vi "p2 - caja fuerte.vi"() -> ()   [LabVIEW 2021]
uses:
  p2 - strongbox.ctl
  p2 - states.ctl
  <vilib>/DAQmx/write.llb/DAQmx Write (Analog DBL 1Chan 1Samp).vi
  <vilib>/DAQmx/read.llb/DAQmx Read (Counter DBL 1Chan 1Samp).vi
  <vilib>/DAQmx/miscellaneous.llb/DAQmx Fill In Error Info.vi
panel:
  in  "stop":bool
  out "turns IRT":dbl format="%0.2f"
  out "turns":i32
  out "direction":bool
  out "password":i32[](array[numeric])
  in  "clean":bool
  in  "unlock":bool
  in  "Knob":i32(knob)=1 scale=1.0..100.0
  out "Boolean":T1
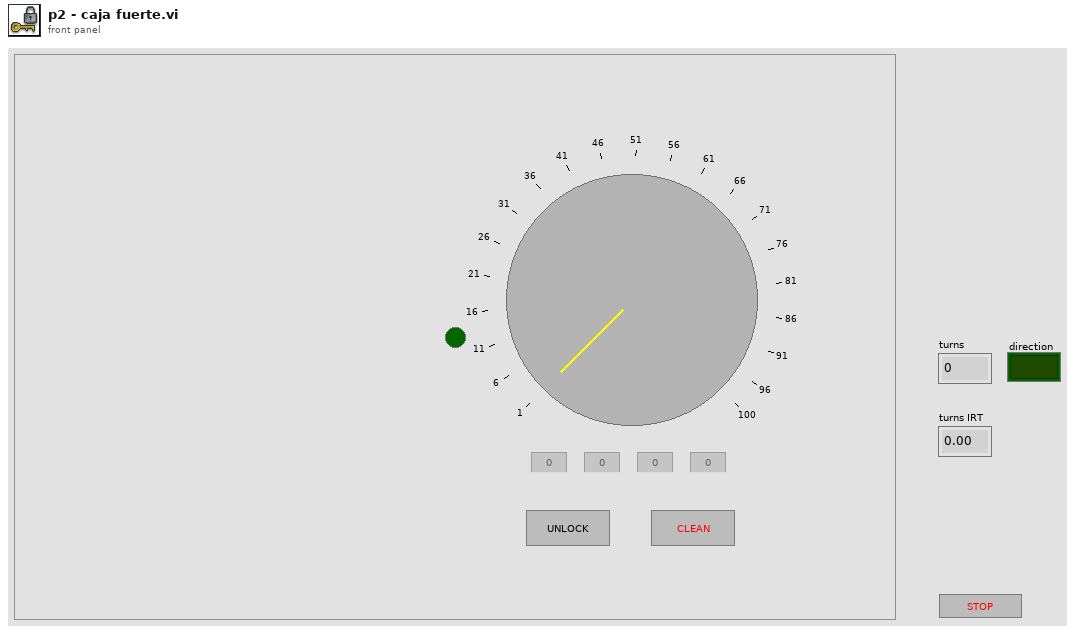
[diagram p1: front panel]
types:
  T1 = typedef "p2 - strongbox.ctl" = bool
  T2 = typedef "p2 - states.ctl" = enum16{"knob", "motor", "animation"}
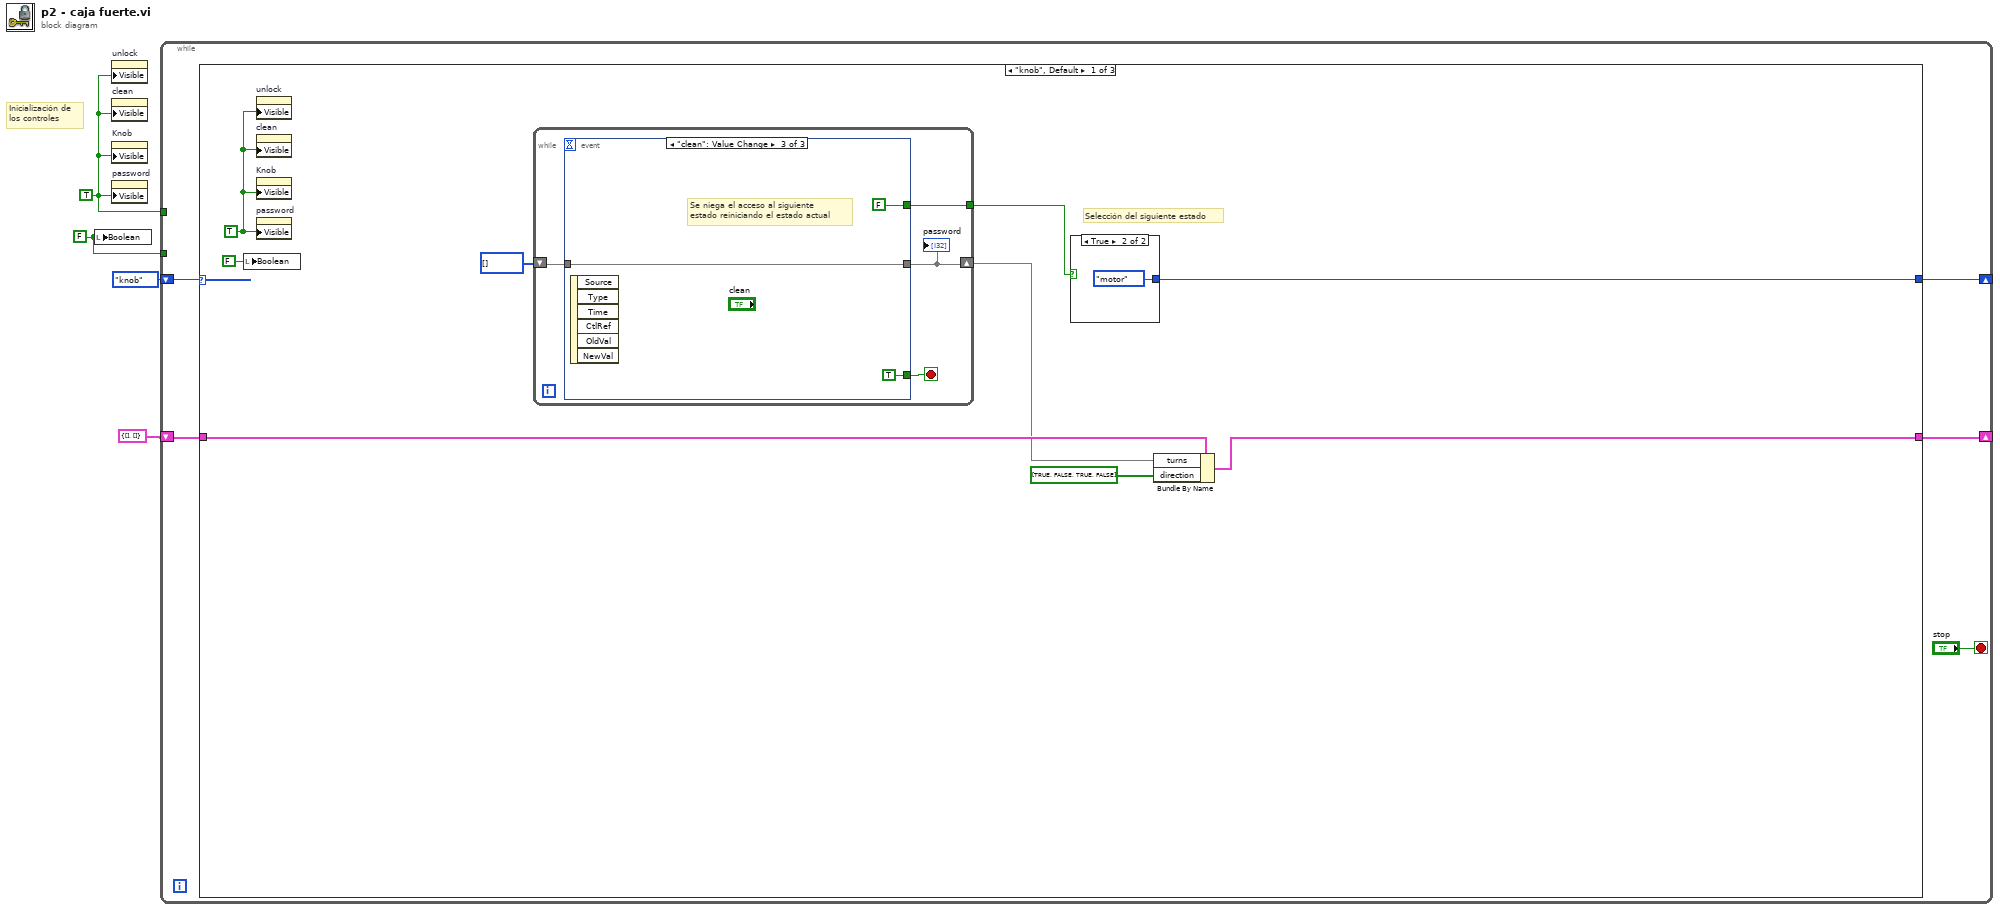
[diagram p0: block diagram]
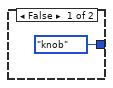
[diagram p2: hidden frame]
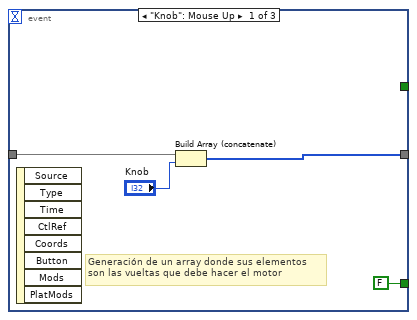
[diagram p3: hidden frame]
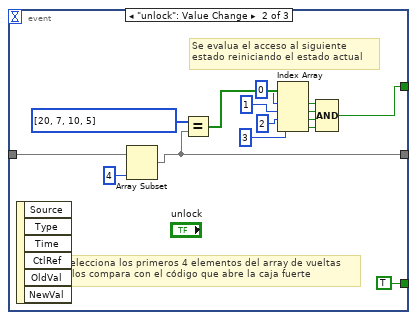
[diagram p4: hidden frame]
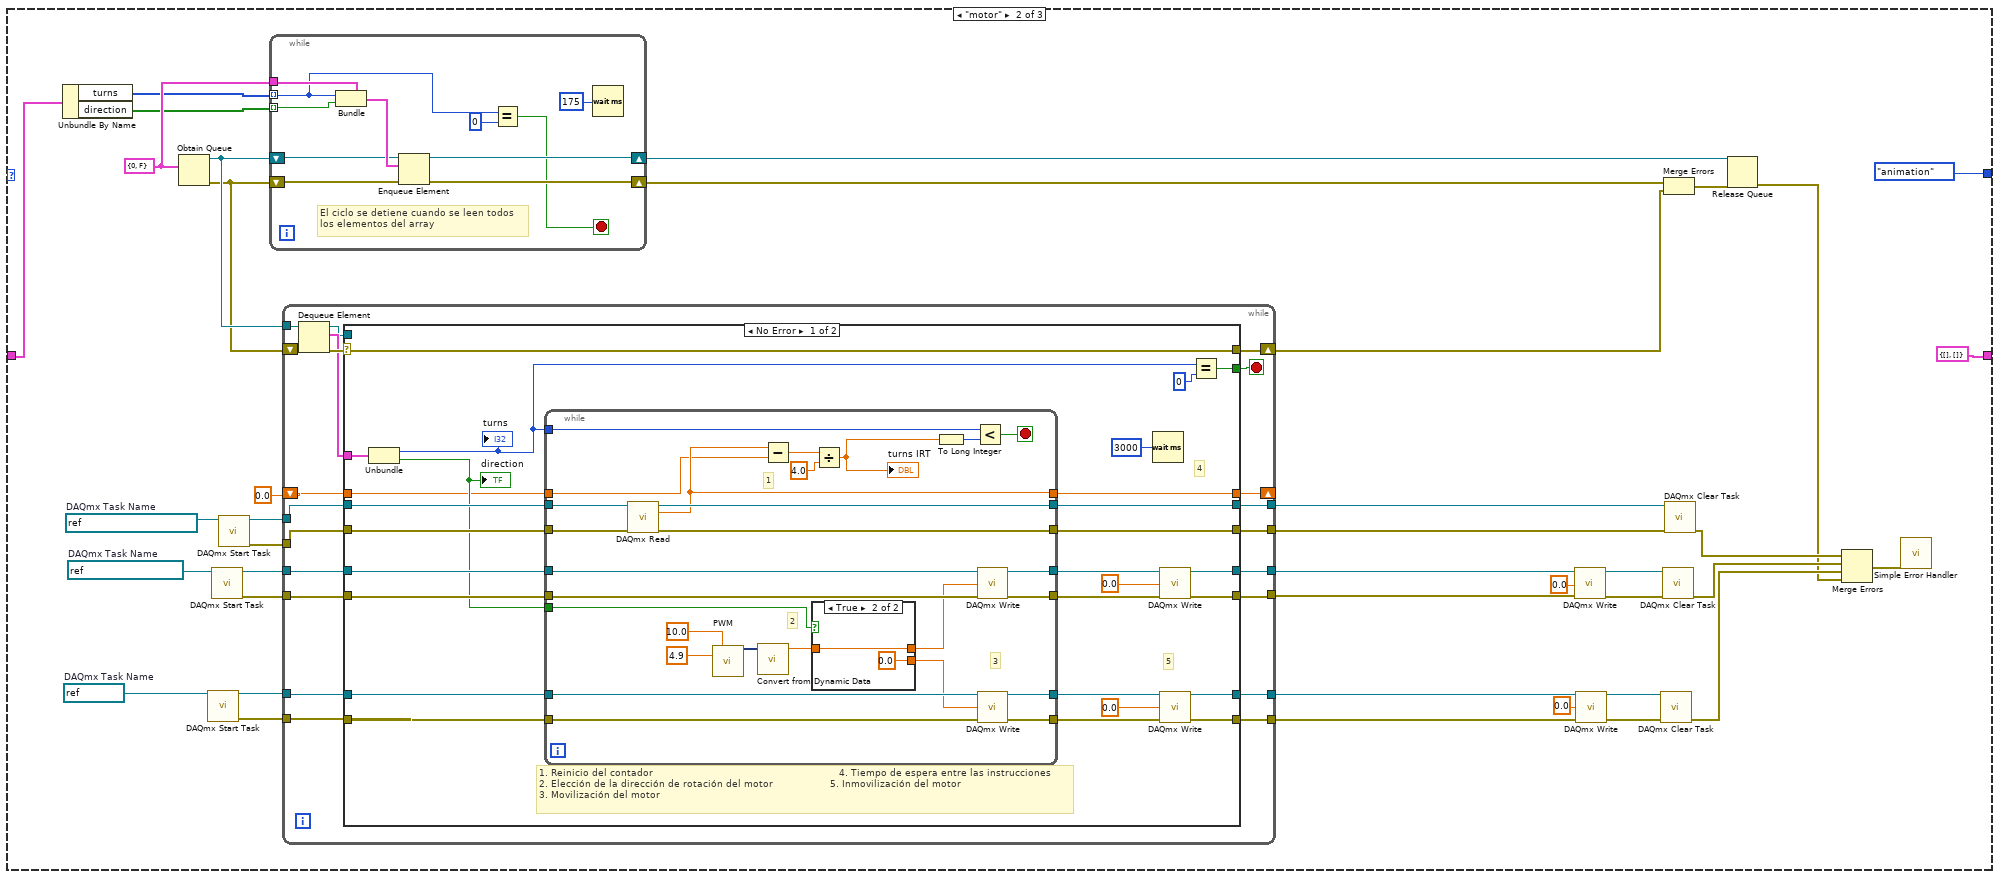
[diagram p5: hidden frame]
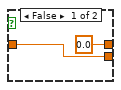
[diagram p6: hidden frame]
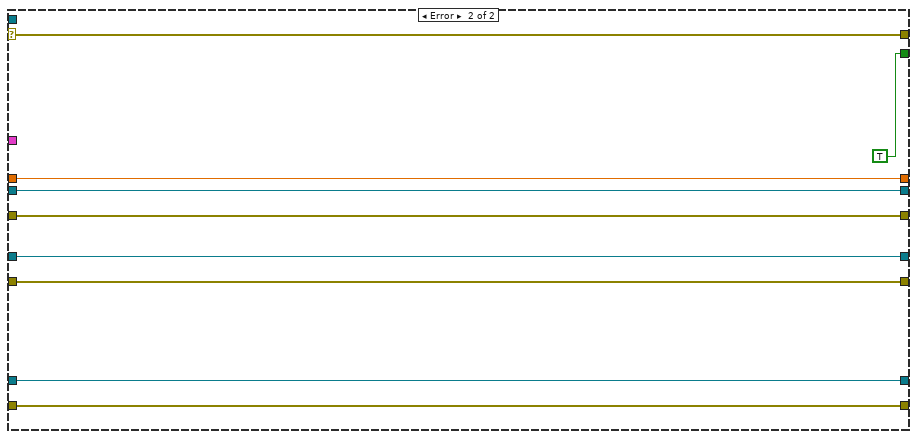
[diagram p7: hidden frame]
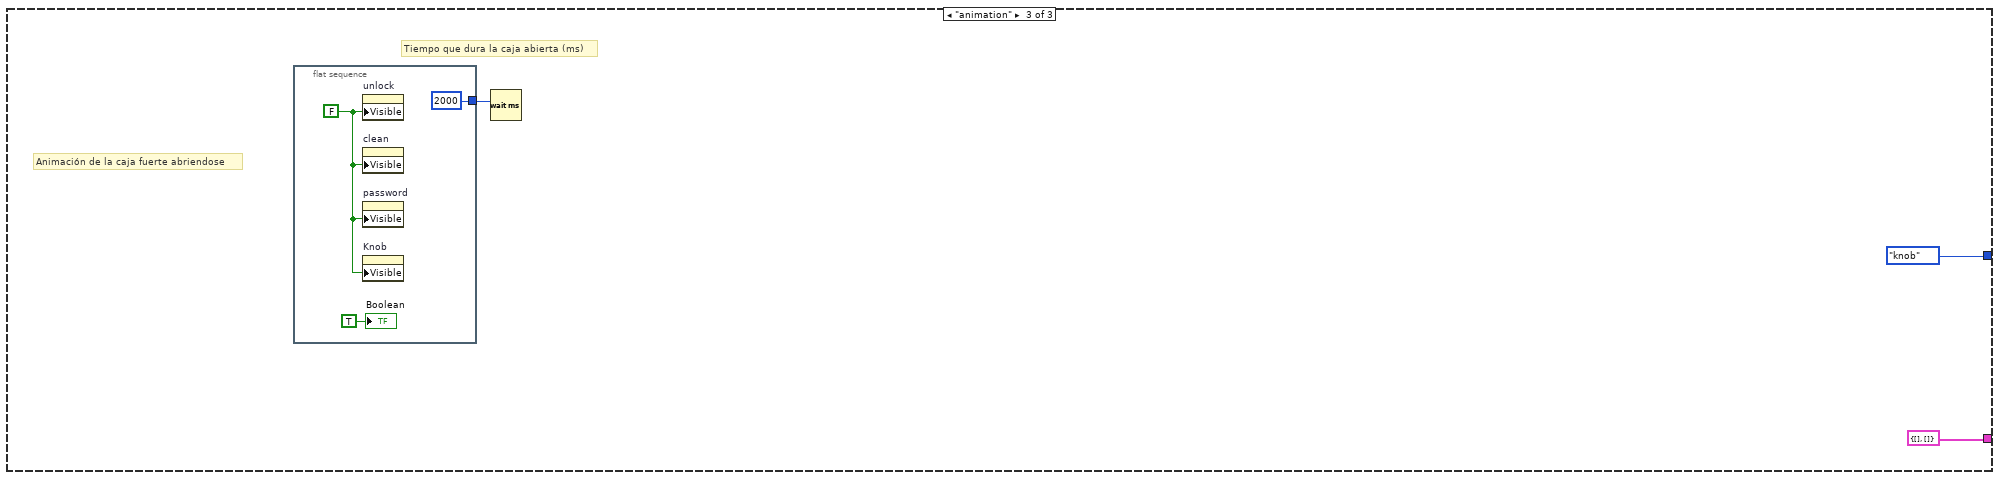
[diagram p8: hidden frame]
diagram:
  w2 = T1 FALSE ("Boolean")
  w1 = TRUE ("Visible")
  # "Inicialización de\nlos controles"
  n1 = local write "Boolean"(w2) -> ()
  n2 = property on="unlock" class="Bool (strict)"("Visible"=w1) -> ()  [unwired: 2 in, 2 out]
  n3 = property on="clean" class="Bool (strict)"("Visible"=w1) -> ()  [unwired: 2 in, 2 out]
  n4 = property on="Knob" class="Knob (strict)"("Visible"=w1) -> ()  [unwired: 2 in, 2 out]
  n5 = property on="password" class="Arr (strict)"("Visible"=w1) -> ()  [unwired: 2 in, 2 out]
  n6 = while {
    shift-right: [w8] -> _
    shift-left: cluster{"turns":i32[], "direction":bool[]} {"turns"=[], "direction"=[]} -> [w9]
    shift-right: [w6] -> _
    shift-left: p2_-_states."knob" -> [w7]
    tunnel: w1 -> [_]
    tunnel: w2 -> [_]
    stop <- "stop" stop-if-true
    n7 = case shown="\"knob\", Default" w7 {
      tunnel: w9 -> [w17 w78 _]
      tunnel: [w16 cluster{"turns":i32[], "direction":bool[]} {"turns"=[], "direction"=[]} cluster{"turns":i32[], "direction":bool[]} {"turns"=[], "direction"=[]}] -> w8
      tunnel: [w15 p2_-_states."animation" p2_-_states."knob"] -> w6
      frame "knob", Default {
        w11 = TRUE ("Visible")
        # "Selección del siguiente estado"
        n8 = local write "Boolean"(T1 FALSE ("Boolean")) -> ()
        n9 = property on="unlock" class="Bool (strict)"("Visible"=w11) -> ()  [unwired: 2 in, 2 out]
        n10 = property on="clean" class="Bool (strict)"("Visible"=w11) -> ()  [unwired: 2 in, 2 out]
        n11 = property on="Knob" class="Knob (strict)"("Visible"=w11) -> ()  [unwired: 2 in, 2 out]
        n12 = property on="password" class="Arr (strict)"("Visible"=w11) -> ()  [unwired: 2 in, 2 out]
        n13 = while {
          shift-right: [w23] -> w13
          shift-left: i32[] [] -> [w24]
          tunnel: [w21] -> w14
          stop <- w22 stop-if-true
          n14 = event shown="[2] \"clean\": Value Change" {
            selector: _ -> [_ _ _]
            dyn-events: _ -> [_ _ _]
            timeout: _ -> [_ _ _]
            tunnel: [w28 w39 w44] -> w23
            tunnel: w24 -> [w27 w40 w44]
            tunnel: [FALSE TRUE TRUE] -> w22
            tunnel: [_ w33 FALSE] -> w21
            event "Knob": Mouse Up {
              # "Generación de un array donde sus elementos\nson las vueltas que debe hacer el motor"
              n15 = event-data() -> ()  [unwired: 1 in, 8 out]
              n16 = Build Array (concatenate)(w27, "Knob") -> (w28:i32[])
            }
            event "unlock": Value Change {
              # "Se evalua el acceso al siguiente estado reiniciando el estado actual"
              # "Selecciona los primeros 4 elementos del array de vueltas\ny los compara con el código que abre la caja fuerte"
              n17 = event-data() -> ()  [unwired: 1 in, 6 out]
              n18 = Array Subset(array=w40, length=4) -> (w39:i32[])  [unwired: 1 in]
              n19 = Equal?(x=i32[] [20, 7, 10, 5], y=w39) -> (x = y?=w38:bool[])
              n20 = Index Array(array=w38, index #1=0 ("index"), index #2=1 ("index"), index #3=2 ("index"), index #4=3 ("index")) -> (element #1=w37:bool, element #2=w36:bool, element #3=w35:bool, element #4=w34:bool)
              n21 = Compound Arithmetic op=AND(w37, w36, w35, w34) -> (w33:bool)
            }
            event "clean": Value Change {
              # "Se niega el acceso al siguiente estado reiniciando el estado actual"
              n22 = event-data() -> ()  [unwired: 1 in, 6 out]
            }
          }
          "password" <- w23
        }
        n23 = case shown="True" w14 {
          tunnel: [p2_-_states."knob" p2_-_states."motor"] -> w15
          frame False {
          }
          frame True {
          }
        }
        n24 = Bundle By Name(cluster=w17, "turns"=w13, "direction"=bool[] [TRUE, FALSE, TRUE, FALSE]) -> (w16:cluster{"turns":i32[], "direction":bool[]})
      }
      frame "motor" {
        w71 = refnum<k21> "Motor"  # DAQmx Task Name
        w72 = refnum<k21> "Motor con PWM"  # DAQmx Task Name
        w73 = refnum<k21> "MyCountEdgesTask"  # DAQmx Task Name
        w84 = cluster{i32, bool} {0, FALSE}
        n25 = Unbundle By Name(w78) -> ("turns"=w77:i32[], "direction"=w76:bool[])
        n26 = Obtain Queue(element data type=w84) -> (queue out=w85:refnum<queue>, error out=w83:errorcluster)  [unwired: 4 in, 1 out]
        n27 = call <vilib>:"DAQmx Start Task.vi"("task/channels in"=w71) -> ("task out"=w65:refnum<k21>, "error out"=w64:errorcluster)  [unwired: 13 in]
        n28 = call <vilib>:"DAQmx Start Task.vi"("task/channels in"=w72) -> ("task out"=w67:refnum<k21>, "error out"=w66:errorcluster)  [unwired: 13 in]
        n29 = call <vilib>:"DAQmx Start Task.vi"("task/channels in"=w73) -> ("task out"=w69:refnum<k21>, "error out"=w68:errorcluster)  [unwired: 13 in]
        n30 = while {
          shift-right: [w179] -> w80
          shift-left: w83 -> [w181]
          shift-right: [w180] -> w81
          shift-left: w85 -> [w182]
          tunnel: w77 -> [w176] mode=indexing
          tunnel: w76 -> [w178] mode=indexing
          tunnel: w84 -> [w177]
          stop <- w174 stop-if-true
          # "El ciclo se detiene cuando se leen todos\nlos elementos del array"
          n31 = Bundle(cluster=w177, w176, w178) -> (w183:cluster{i32, bool})
          n32 = Enqueue Element(queue=w182, element=w183, error in (no error)=w181) -> (queue out=w180:refnum<queue>, error out=w179:errorcluster)  [unwired: 1 in, 1 out]
          n33 = Equal?(x=w176, y=0) -> (x = y?=w174:bool)
          n34 = Wait (ms)(milliseconds to wait=u32 175) -> ()  [unwired: 1 out]
        }
        n35 = while {
          tunnel: w85 -> [w106]
          shift-right: [w102] -> w82
          shift-left: w83 -> [w103]
          tunnel: w69 -> [w98]
          tunnel: w68 -> [w99]
          tunnel: w67 -> [w95]
          tunnel: w66 -> [w93]
          tunnel: [w97] -> w53
          tunnel: [w96] -> w52
          tunnel: [w94] -> w51
          tunnel: [w92] -> w50
          tunnel: w65 -> [w91]
          tunnel: w64 -> [w90]
          tunnel: [w89] -> w49
          tunnel: [w88] -> w48
          shift-right: [w86] -> _
          shift-left: 0.0 ("data") -> [w87]
          stop <- w101 stop-if-true
          n36 = Dequeue Element(queue=w106, error in (no error)=w103) -> (queue out=w100:refnum<queue>, element=w104:cluster{i32, bool}, error out=w105:errorcluster)  [unwired: 1 in, 1 out]
          n37 = case shown="No Error" w105 {
            selector: w105 -> [w132 w172]
            tunnel: w104 -> [w133 _]
            tunnel: [w130 TRUE] -> w101
            tunnel: [w132 w172] -> w102
            tunnel: w100 -> [_ _]
            tunnel: w99 -> [w128 w170]
            tunnel: w98 -> [w129 w171]
            tunnel: [w123 w171] -> w97
            tunnel: [w122 w170] -> w96
            tunnel: [w116 w169] -> w94
            tunnel: w95 -> [w127 w169]
            tunnel: w93 -> [w126 w168]
            tunnel: [w115 w168] -> w92
            tunnel: w91 -> [w125 w167]
            tunnel: w90 -> [w124 w166]
            tunnel: [w111 w167] -> w89
            tunnel: [w110 w166] -> w88
            tunnel: w87 -> [w120 w165]
            tunnel: [w119 w165] -> w86
            frame No Error {
              # "5"
              # "4"
              # "1. Reinicio del contador                                                              4. Tiempo de espera entre las instrucciones\n2. Elección de la dirección de rotación del motor                   5. Inmovilización del motor \n3. Movilización del motor"
              n38 = Unbundle(w133) -> (w118:i32, w121:bool)
              "turns" <- w118
              "direction" <- w121
              n39 = while {
                tunnel: w129 -> [w160]
                tunnel: [w158] -> w123
                tunnel: w128 -> [w159]
                tunnel: [w157] -> w122
                tunnel: [w155] -> w119
                tunnel: w120 -> [w154]
                tunnel: w127 -> [w150]
                tunnel: w126 -> [w149]
                tunnel: [w148] -> w117
                tunnel: [w147] -> w114
                tunnel: w125 -> [w143]
                tunnel: w124 -> [w142]
                tunnel: [w141] -> w113
                tunnel: [w140] -> w112
                tunnel: w121 -> [w139]
                tunnel: w118 -> [w134]
                stop <- w135 stop-if-true
                # "3"
                # "2"
                # "1"
                n40 = call-poly <vilib>:"DAQmx Read.vi"("task/channels in"=w160, "error in"=w159) -> ("task out"=w158:refnum<k21>, "data"=w155:dbl, "error out"=w157:errorcluster)  [unwired: 11 in]
                n41 = call "PWM"("Duty Cycle (%)"=10.0, "Frequency"=4.9) -> ("Square"=w153:dynamicdata)  [unwired: 12 in, 1 out]
                n42 = call "Convert from Dynamic Data"("Dynamic Data Type"=w153) -> ("Scalar"=w136:dbl)  [unwired: 3 in]
                n43 = Subtract(x=w155, y=w154) -> (x-y=w146:dbl)
                n44 = case shown="True" w139 {
                  tunnel: [w161 0.0] -> w138
                  tunnel: [0.0 w163] -> w137
                  tunnel: w136 -> [w161 w163]
                  frame False {
                  }
                  frame True {
                  }
                }
                n45 = Divide(x=w146, y=4.0) -> (x/y=w144:dbl)
                "turns IRT" <- w144
                n46 = To Long Integer(number=w144) -> (32bit integer=w156:i32)
                n47 = Less?(x=w134, y=w156) -> (x < y?=w135:bool)
                n48 = call-poly <vilib>:"DAQmx Write.vi"("task/channels in"=w150, "data"=w137, "error in"=w149) -> ("task out"=w148:refnum<k21>, "error out"=w147:errorcluster)  [unwired: 10 in, 1 out]
                n49 = call-poly <vilib>:"DAQmx Write.vi"("task/channels in"=w143, "data"=w138, "error in"=w142) -> ("task out"=w141:refnum<k21>, "error out"=w140:errorcluster)  [unwired: 10 in, 1 out]
              }
              n50 = Wait (ms)(milliseconds to wait=u32 3000) -> ()  [unwired: 1 out]
              n51 = call-poly <vilib>:"DAQmx Write.vi"("task/channels in"=w117, "data"=0.0, "error in"=w114) -> ("task out"=w116:refnum<k21>, "error out"=w115:errorcluster)  [unwired: 10 in, 1 out]
              n52 = call-poly <vilib>:"DAQmx Write.vi"("task/channels in"=w113, "data"=0.0, "error in"=w112) -> ("task out"=w111:refnum<k21>, "error out"=w110:errorcluster)  [unwired: 10 in, 1 out]
              n53 = Equal?(x=w118, y=0) -> (x = y?=w130:bool)
            }
            frame Error {
            }
          }
        }
        n54 = call-poly <vilib>:"DAQmx Write.vi"("task/channels in"=w51, "data"=0.0, "error in"=w50) -> ("task out"=w62:refnum<k21>, "error out"=w58:errorcluster)  [unwired: 10 in, 1 out]
        n55 = call-poly <vilib>:"DAQmx Write.vi"("task/channels in"=w49, "data"=0.0, "error in"=w48) -> ("task out"=w56:refnum<k21>, "error out"=w57:errorcluster)  [unwired: 10 in, 1 out]
        n56 = call <vilib>:"DAQmx Clear Task.vi"("task in"=w56, "error in"=w57) -> ("error out"=w55:errorcluster)  [unwired: 13 in]
        n57 = call <vilib>:"DAQmx Clear Task.vi"("task in"=w62, "error in"=w58) -> ("error out"=w60:errorcluster)  [unwired: 13 in]
        n58 = Merge Errors(w80, w82) -> (w79:errorcluster)
        n59 = call <vilib>:"DAQmx Clear Task.vi"("task in"=w53, "error in"=w52) -> ("error out"=w61:errorcluster)  [unwired: 13 in]
        n60 = Release Queue(queue=w81, error in (no error)=w79) -> (error out=w47:errorcluster)  [unwired: 1 in, 2 out]
        n61 = Merge Errors(w61, w60, w55, w47) -> (w59:errorcluster)
        n62 = call <vilib>:"Simple Error Handler.vi"("error in (no error)"=w59) -> ()  [unwired: 4 in, 5 out]
      }
      frame "animation" {
        # "Tiempo que dura la caja abierta (ms)"
        # "Animación de la caja fuerte abriendose"
        n63 = flat-sequence {
          tunnel: [u32 2000 ("milliseconds to wait")] -> w185
          frame #0 {
            w189 = FALSE ("Visible")
            n64 = property on="unlock" class="Bool (strict)"("Visible"=w189) -> ()  [unwired: 2 in, 2 out]
            n65 = property on="clean" class="Bool (strict)"("Visible"=w189) -> ()  [unwired: 2 in, 2 out]
            n66 = property on="password" class="Arr (strict)"("Visible"=w189) -> ()  [unwired: 2 in, 2 out]
            n67 = property on="Knob" class="Knob (strict)"("Visible"=w189) -> ()  [unwired: 2 in, 2 out]
            "Boolean" <- T1 TRUE ("Boolean")
          }
        }
        n68 = Wait (ms)(milliseconds to wait=w185) -> ()  [unwired: 1 out]
      }
    }
  }
